vi "Scale LabVIEW PSD with central frequency and reference level info.vi"(8 "error in (no error)":errorcluster, 9 "Reference level":dbl, 10 "Central frequency":dbl, 11 "Power Spectrum / PSD in":cluster{"f0":dbl, "df":dbl, "magnitude":dbl[]}) -> (0 "error out":errorcluster, 3 "Power Spectrum / PSD out":cluster{"f0":dbl, "df":dbl, "magnitude":dbl[]})   [LabVIEW 2020]
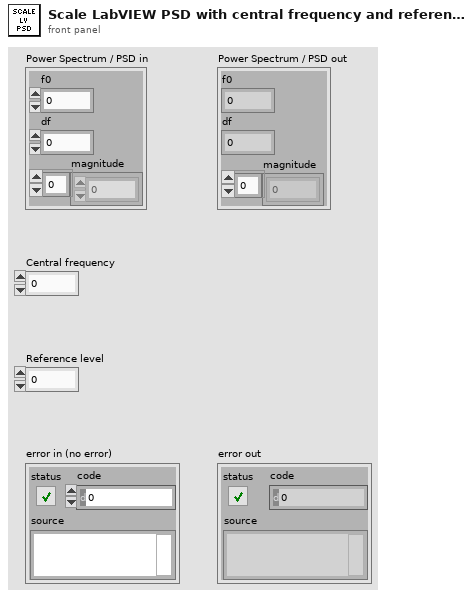
[diagram p1: front panel]
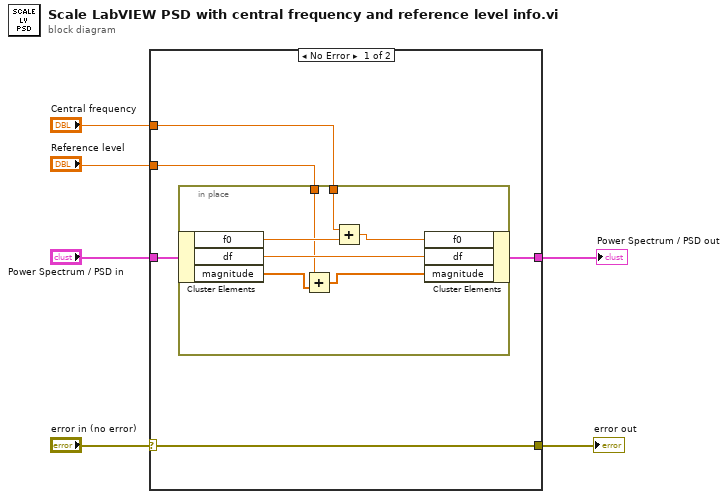
[diagram p0: block diagram]
diagram:
  n1 = case shown="No Error" "error in (no error)" {
    selector: "error in (no error)" -> [w11 w20]
    tunnel: [w7 w19] -> w6
    tunnel: "Power Spectrum / PSD in" -> [w10 w19]
    tunnel: "Central frequency" -> [w9 _]
    tunnel: [w11 w20] -> w2
    tunnel: "Reference level" -> [w8 _]
    frame No Error {
      n2 = in-place {
        in-place-border: w9 -> [w17]
        in-place-border: w8 -> [w13]
        n3 = in-place-cluster #1(w10) -> ("f0"=w18:dbl, "df"=w15:dbl, "magnitude"=w14:dbl[])
        n4 = Add(x=w13, y=w14) -> (x+y=w12:dbl[])
        n5 = Add(x=w17, y=w18) -> (x+y=w16:dbl)
        n6 = in-place-cluster #1("f0"=w16, "df"=w15, "magnitude"=w12) -> (w7:cluster{"f0":dbl, "df":dbl, "magnitude":dbl[]})
      }
    }
    frame Error {
    }
  }
  "Power Spectrum / PSD out" <- w6
  "error out" <- w2
